vi "Read 568x with Auto-Averaging.vi"(0 "reference":refnum<k15>, 5 "Frequency (Hz)":dbl, 11 "error in (no error)":errorcluster, 12 "Total Aperture Time Limit (s)":dbl=120.0 format="%#_13g", 14 "Maximum Two Sigma Uncertainty (dB)":dbl=0.05 format="%#_13g") -> (4 "reference out":refnum<k15>, 6 "measurement":dbl, 15 "error out":errorcluster)   [LabVIEW 2023, in "NI-568x RF Power Meter.lvlib" / "SG 2250 Path Accessor.lvclass"]
uses:
  SG 2250 Path Accessor.lvclass
  <instrlib>/ni568x/ni568x.llb/ni568x Read.vi
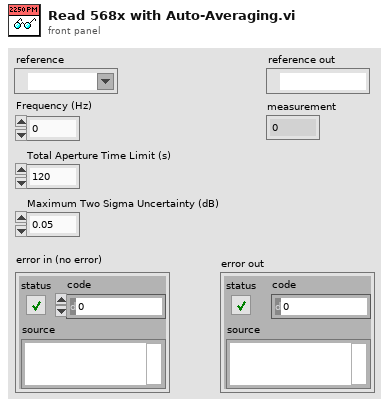
[diagram p1: front panel]
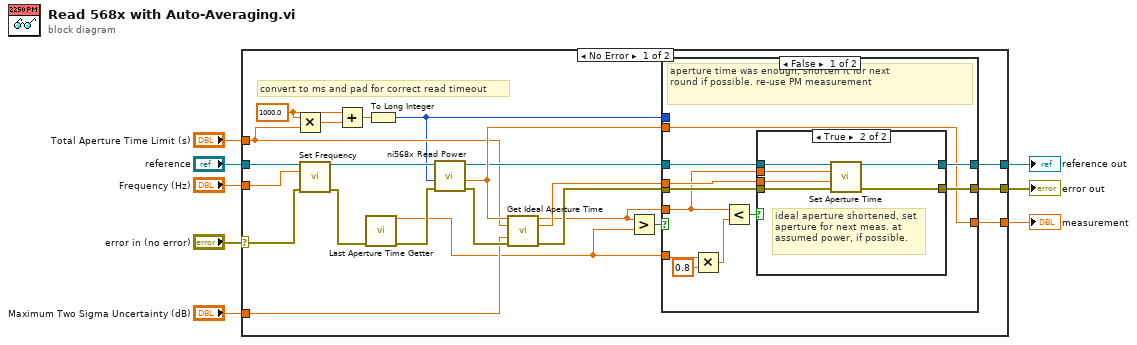
[diagram p0: block diagram]
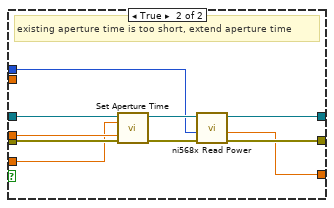
[diagram p3: hidden frame]
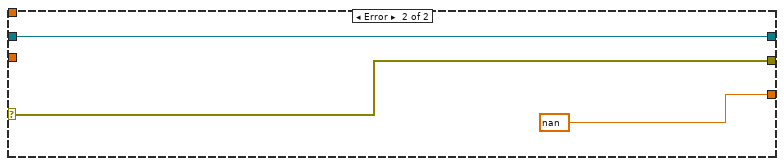
[diagram p4: hidden frame]
diagram:
  n1 = case shown="No Error" "error in (no error)" {
    selector: "error in (no error)" -> [w27 w62]
    tunnel: [w30 w62] -> w7
    tunnel: "reference" -> [w25 w63]
    tunnel: [w29 w63] -> w3
    tunnel: [w28 nan ("Power(dBm)")] -> w6
    tunnel: "Frequency (Hz)" -> [w24 _]
    tunnel: "Total Aperture Time Limit (s)" -> [w12 _]
    tunnel: "Maximum Two Sigma Uncertainty (dB)" -> [w15 _]
    frame No Error {
      w10 = 1000.0 ("x")
      # "convert to ms and pad for correct read timeout"
      n2 = Multiply(x=w10, y=w12) -> (x*y=w13:dbl)
      n3 = call "Set Frequency.vi"("reference"=w25, "Frequency (Hz)"=w24, "error in (no error)"=w27) -> ("reference out"=w21:refnum<k15>, "error out"=w26:errorcluster)  [unwired: 11 in]
      n4 = Add(x=w10, y=w13) -> (x+y=w11:dbl)
      n5 = call "Last Aperture Time Getter.vi"("error in (no error)"=w26) -> ("Aperture Time (s)"=w14:dbl, "error out"=w22:errorcluster)  [unwired: 13 in]
      n6 = To Long Integer(number=w11) -> (32bit integer=w9:i32)
      n7 = call-poly <instrlib>:"ni568x Read Power.vi"("error in"=w22, "maximum time (5000ms)"=w9, "instrument handle"=w21) -> ("error out"=w23:errorcluster, "power"=w20:dbl, "instrument handle out"=w18:refnum<k15>)  [unwired: 6 in]
      n8 = call "Get Ideal Aperture Time.vi"("Measured Power (dBm)"=w20, "Total Aperture Time Limit (s)"=w12, "Maximum Two Sigma Uncertainty (dB)"=w15, "error in (no error)"=w23) -> ("Ideal Total Aperture time (s)"=w16:dbl, "Ideal Number of Averages"=w17:dbl, "error out"=w19:errorcluster)  [unwired: 9 in]
      n9 = Greater?(x=w16, y=w14) -> (0:w31:bool)
      n10 = case shown="False" w31 {
        tunnel: w16 -> [w32 w51]
        tunnel: w14 -> [w42 _]
        tunnel: [w40 w58] -> w30
        tunnel: [w39 w59] -> w29
        tunnel: [w37 w56] -> w28
        tunnel: w20 -> [w37 _]
        tunnel: w19 -> [w35 w55]
        tunnel: w17 -> [w33 w53]
        tunnel: w18 -> [w36 w54]
        tunnel: w9 -> [_ w52]
        frame False {
          # "aperture time was enough, shorten it for next\nround if possible. re-use PM measurement"
          n11 = Multiply(x=w42, y=0.8 ("aperture shrink hysteresis factor")) -> (x*y=w41:dbl)
          n12 = Less?(x=w32, y=w41) -> (x < y?=w38:bool)
          n13 = case shown="True" w38 {
            tunnel: [w44 w50] -> w40
            tunnel: [w43 w46] -> w39
            tunnel: w36 -> [w43 w49]
            tunnel: w35 -> [w44 w48]
            tunnel: w32 -> [_ w47]
            tunnel: w33 -> [_ w45]
            frame False {
            }
            frame True {
              # "ideal aperture shortened, set\naperture for next meas. at\nassumed power, if possible."
              n14 = call "Set Aperture Time.vi"("reference"=w49, "Aperture Time(s)"=w47, "Number of Averages"=w45, "error in (no error)"=w48) -> ("reference out"=w46:refnum<k15>, "error out"=w50:errorcluster)  [unwired: 10 in]
            }
          }
        }
        frame True {
          # "existing aperture time is too short, extend aperture time"
          n15 = call "Set Aperture Time.vi"("reference"=w54, "Aperture Time(s)"=w51, "Number of Averages"=w53, "error in (no error)"=w55) -> ("reference out"=w60:refnum<k15>, "error out"=w57:errorcluster)  [unwired: 10 in]
          n16 = call-poly <instrlib>:"ni568x Read Power.vi"("error in"=w57, "maximum time (5000ms)"=w52, "instrument handle"=w60) -> ("error out"=w58:errorcluster, "power"=w56:dbl, "instrument handle out"=w59:refnum<k15>)  [unwired: 6 in]
        }
      }
    }
    frame Error {
    }
  }
  "error out" <- w7
  "measurement" <- w6
  "reference out" <- w3
